vi "PR Check Voltage Of Pulser.vi"(1 "VoltLevel":i32) -> (0 "Normal":bool)   [LabVIEW 2022 SP3, in "BS6006PRPLUS.lvlib"]
uses:
  BS6006PRPLUS.lvlib
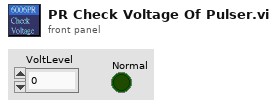
[diagram p1: front panel]
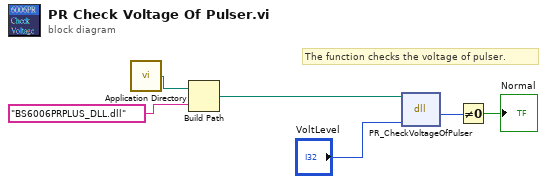
[diagram p0: block diagram]
diagram:
  # "The function checks the voltage of pulser."
  n1 = call <vilib>:"Application Directory.vi"() -> ("Application Directory"=w3:path)
  n2 = Build Path(base path=w3, name or relative path="BS6006PRPLUS_DLL.dll") -> (appended path=w1:path)
  n3 = dll-call lib="E:/Broadsound_Program/PulserReceiver/6006PR PLUS/API/DLL/LabVIEW 15/VIs/BS6006PRPLUS_DLL.dlls" fn="PR_CheckVoltageOfPulser"(path in=w1, "VoltLevel"="VoltLevel") -> ("Normal"=w5:u8)  [unwired: 3 in, 2 out]
  n4 = Not Equal To 0?(x=w5) -> (x != 0?=→"Normal":bool)
